vi "uploadSettingsToCamera.vi"(8 "error in (no error)":errorcluster, 10 "Path":path, 11 "CameraManager in":refnum<class "CameraManager.lvclass">) -> (0 "error out":errorcluster, 3 "CameraManager out":refnum<class "CameraManager.lvclass">)   [LabVIEW 2011, in "iManagement.lvlib" / "CameraManager.lvclass"]
doc: "Upload the settings to the camera."
uses:
  CameraManager.lvclass
  CameraManager.lvclass/CameraManager.ctl
  Hal/Channels/Camera/CameraController.lvclass
  Hal/Channels/Camera/CameraEventsManager/CameraEventsManger.lvclass
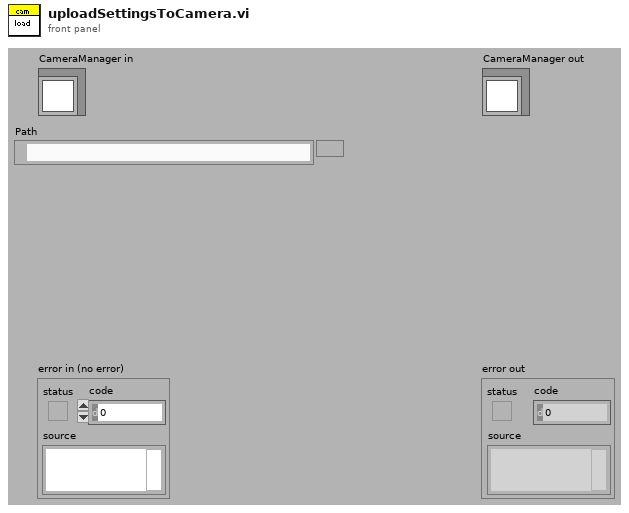
[diagram p1: front panel]
types:
  T1 = cluster{"loadCameraSettingsEvent":refnum<user-event>}
  T2 = cluster{"settingsFrontEndEvents":cluster{"loadSettingsFromPath":refnum<user-event>, "lookUpElementEvent":refnum<user-event>, "saveSettings":refnum<user-event>, "loadSettings":refnum<user-event>, "close":refnum<user-event>, "replaceElement":refnum<user-event>, "findParentNodes":refnum<user-event>, "createNode":refnum<user-event>}, "settingBackEndEvents":cluster{"defaultSettingsPathRequest":refnum<user-event>, "searchResultEvent":refnum<user-event>, "settingsSaved":refnum<user-event>, "settingsLoaded":refnum<user-event>, "foundParentNode":refnum<user-event>}}
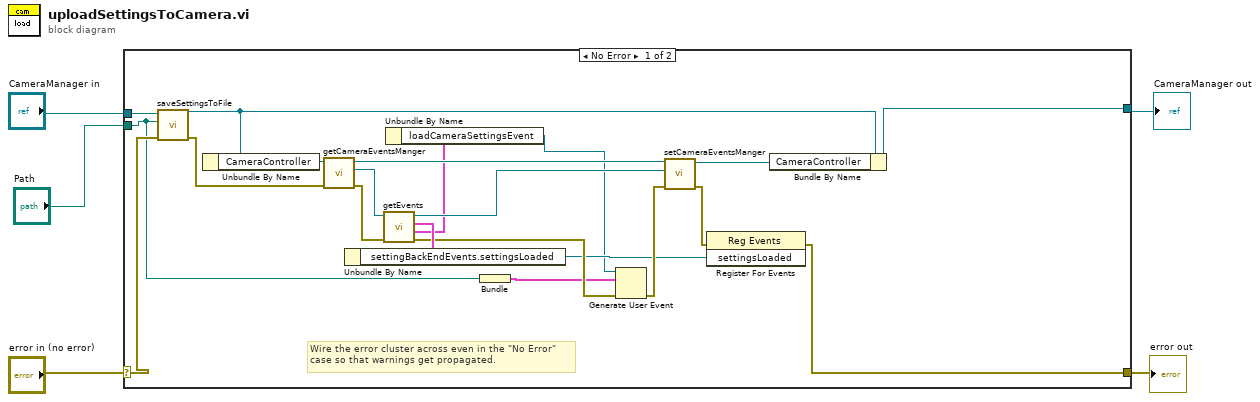
[diagram p0: block diagram]
diagram:
  # "Wire the error cluster across even in the \"No Error\"\ncase so that warnings get propagated."
  n1 = case shown="No Error" "error in (no error)" {
    selector: "error in (no error)" -> [w14 w28]
    tunnel: [w10 w28] -> w2
    tunnel: [w21 w27] -> w3
    tunnel: "CameraManager in" -> [w16 w27]
    tunnel: "Path" -> [w6 _]
    frame No Error {
      n2 = call "saveSettingsToFile.vi"("error in (no error)"=w14, "Path"=w6, "CameraManager in"=w16) -> ("error out"=w13:errorcluster, "CameraManager out"=w15:refnum<class "CameraManager.lvclass">)  [unwired: 7 in]
      n3 = Unbundle By Name(w15) -> ("CameraController"=w24:refnum<class "CameraController.lvclass">)
      n4 = call-dynamic "getCameraEventsManger.vi"("error in (no error)"=w13, "CameraController.lvclass in"=w24) -> ("error out"=w25:errorcluster, "Hardware:Channels.lvlib:CameraEventsManger.lvclass"=w26:refnum<class "CameraEventsManger.lvclass">, "CameraController.lvclass out"=w23:refnum<class "CameraController.lvclass">)  [unwired: 7 in]
      n5 = call-dynamic "getEvents.vi"("error in (no error)"=w25, "CameraEventsManger in"=w26) -> ("error out"=w18:errorcluster, "cameraSettingsEventsRef"=w9:T1, "settingsEvents"=w19:T2, "CameraEventsManger out"=w20:refnum<class "CameraEventsManger.lvclass">)  [unwired: 5 in, 1 out]
      n6 = Unbundle By Name(w19) -> ("settingBackEndEvents.settingsLoaded"=w12:refnum<user-event>)
      n7 = Unbundle By Name(w9) -> ("loadCameraSettingsEvent"=w8:refnum<user-event>)
      n8 = Bundle("Path"=w6) -> (w7:cluster{"Path":path})  [unwired: 1 in]
      n9 = Generate User Event(user event=w8, event data cluster=w7, error in=w18) -> (error out=w17:errorcluster)  [unwired: 1 out]
      n10 = call-dynamic "setCameraEventsManger.vi"("error in (no error)"=w17, "Hardware:Channels.lvlib:CameraEventsManger.lvclass"=w20, "CameraController.lvclass in"=w23) -> ("error out"=w11:errorcluster, "CameraController.lvclass out"=w22:refnum<class "CameraController.lvclass">)  [unwired: 7 in]
      n11 = register-events(error in=w11, w12) -> (error out=w10:errorcluster)  [unwired: 1 in, 1 out]
      n12 = Bundle By Name(cluster=w15, "CameraController"=w22) -> (w21:refnum<class "CameraManager.lvclass">)
    }
    frame Error {
    }
  }
  "error out" <- w2
  "CameraManager out" <- w3
